vi "Build lookup key for configuration.vi"(8 "error in (no error)":errorcluster, 11 "Modbus Module configuration in":refnum<class "Modbus Module configuration.lvclass">) -> (0 "error out":errorcluster, 1 "ok?":bool, 2 "key":string, 3 "Modbus Module configuration out":refnum<class "Modbus Module configuration.lvclass">)   [LabVIEW 2015, in "Modbus Module runtime.lvclass"]
uses:
  <vilib>/NI/DCAF/Modules/modbus/module/execution/Modbus Module runtime.lvclass
  <vilib>/NI/DCAF/Modules/modbus/module/configuration/Modbus Module configuration.lvclass
  <vilib>/NI/DCAF/Modules/modbus/module/configuration/Modbus Module configuration.lvclass/Modbus Module configuration.ctl
  <vilib>/NI/DCAF/Modules/modbus/module/configuration/Read class.vi
  <vilib>/NI/DCAF/Modules/modbus/module/configuration/Read VISA resource name.vi
  <vilib>/NI/DCAF/Modules/modbus/module/configuration/Read IP address.vi
  <vilib>/NI/DCAF/Modules/modbus/module/configuration/Read port (502).vi
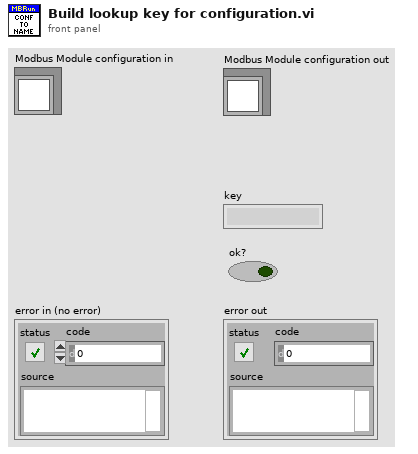
[diagram p1: front panel]
types:
  T1 = typedef "Modbus Slave configuration.lvclass/modbus class.ctl" = enum16{"TCP master", "TCP slave", "serial master", "serial slave"}
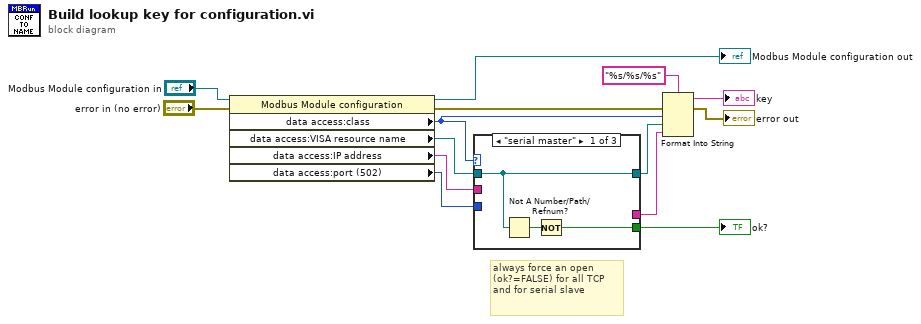
[diagram p0: block diagram]
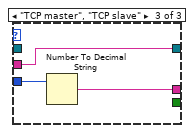
[diagram p3: hidden frame]
diagram:
  # "always force an open (ok?=FALSE) for all TCP and for serial slave"
  n1 = property class="Modbus Module configuration"(reference="Modbus Module configuration in", error in="error in (no error)") -> (reference out=→"Modbus Module configuration out":refnum<class "Modbus Module configuration.lvclass">, error out=w9:errorcluster, "data access:class"=w5:T1, "data access:VISA resource name"=w6:refnum<visa-resource-name>, "data access:IP address"=w12:string, "data access:port (502)"=w8:u16)
  n2 = case shown="\"serial master\"" w5 {
    tunnel: w6 -> [w17 w18 _]
    tunnel: [w17 w18 w19] -> w7
    tunnel: w8 -> [_ _ w21]
    tunnel: [w15 _ _] -> w13
    tunnel: [_ _ w20] -> w11
    tunnel: w12 -> [_ _ w19]
    frame "serial master" {
      n3 = Not A Number/Path/Refnum?(number/path/refnum=w17) -> (NaN/Path/Refnum?=w16:bool)
      n4 = Not(x=w16) -> (.not. x?=w15:bool)
    }
    frame "serial slave" {
    }
    frame "TCP master", "TCP slave" {
      n5 = Number To Decimal String(number=w21) -> (decimal integer string=w20:string)  [unwired: 1 in]
    }
  }
  "ok?" <- w13
  n6 = Format Into String(format string="%s/%s/%s", error in=w9, w5, w7, w11) -> (resulting string=→"key":string, error out=→"error out":errorcluster)  [unwired: 1 in]
